vi "2021 Advent puzzle 03b.vi"() -> ()   [LabVIEW 2021]
panel:
  out "x*y":u64
  out "subarray":bool[](array[boolean])
  out "Boolean array 2":bool[][](array[boolean])
  out "number 2":u32
  out "column length 2":i32
  out "Array 2":bool[][](array[boolean])
  out "number":u32
  out "Boolean array":bool[][](array[boolean])
  out "transposed array":bool[][](array[boolean])
  out "Array":bool[][](array[boolean])
  out "Width":i32
  out "column length":i32
  # "11110, 10110, 10111, 10101, 11100, 10000, and 11001."
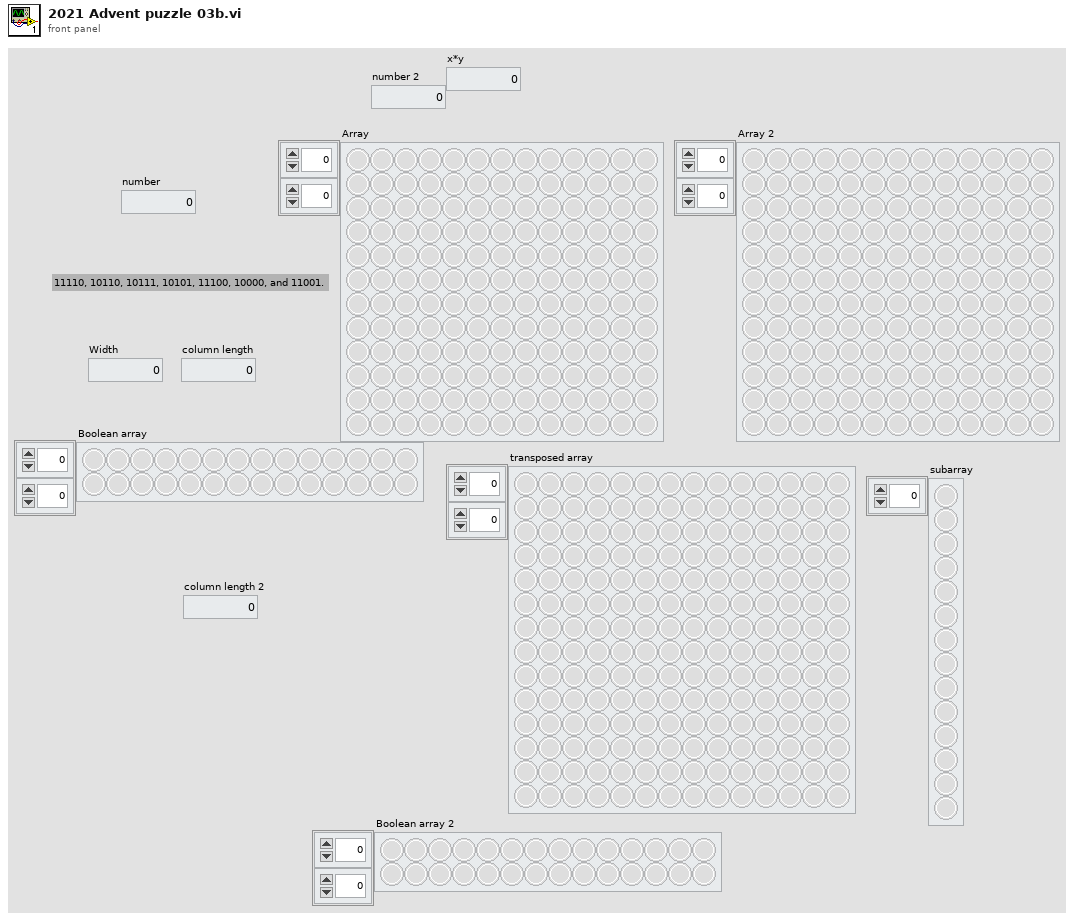
[diagram p1: front panel]
diagram:
  (unwired) "00100\n11110\n10110\n10111\n10101\n01111\n00111\n11100\n10000\n11001\n00010\n01010"
  w6 = "000001100010\n100111011010\n001100011001\n011010001010\n011010101011\n001001110101\n100110001101\n100010010011\n011110000110\n011000110110\n011111111110\n100111110011\n110000100101\n011010011111\n001010011101\n110110001010\n101111110101\n000010101101\n111010111110\n111110001110\n100110111011\n101011010101\n001001000101\n111101000100\n001100000010\n010001100101\n001010011111\n101010010100\n100001110011\n100000111010\n100101010101\n000000101000\n011010100011\n110100111110\n010010011000\n000101000010\n001100011100\n011101000000\n010110111010\n101101100100\n000000010011\n000101001111\n011011100111\n101111100101\n101001101011\n101100010100\n00..."
  # "calc number of 1s per original column\n(number > ((column length div 2 ))generates a true"
  # "determine the number of bits er line"
  n1 = Spreadsheet String To Array(delimiter (Tab)="\n", format string="%b", spreadsheet string=w6, array type (2D Dbl)=i32[] []) -> (array=w14:i32[])
  n2 = Scan From String(format string="%s", input string=w6) -> (output 1=w15:string)  [unwired: 3 in, 3 out]
  n3 = for {
    tunnel: w14 -> [w21] mode=indexing
    tunnel: [w20] -> w11 mode=indexing
    n4 = Number To Boolean Array(number=w21) -> (Boolean array=w20:bool[])
  }
  "transposed array" <- w11
  n5 = String Length(string=w15) -> (length=w7:i32)
  "Width" <- w7
  n6 = Decrement(x=w7) -> (x-1=w8:i32)
  n7 = for {
    N: w7 -> [_]
    shift-right: [w27] -> w13
    shift-left: w11 -> [w28]
    tunnel: w8 -> [w30]
    i -> [w26]
    stop <- w25 stop-if-true
    n8 = Subtract(x=w30, y=w26) -> (x-y=w29:i32)
    n9 = Matrix Size(0:w28) -> (1:w35:i32)  [unwired: 1 out]
    "column length" <- w35
    n10 = Index Array(array=w28, index (col)=w29) -> (element=w31:bool[])  [unwired: 1 in]
    n11 = Boolean To (0,1)(Boolean=w31) -> (0, 1=w32:i16[])
    n12 = Add Array Elements(numeric array=w32) -> (sum=w36:i16)
    n13 = Divide(x=w35, y=2) -> (x/y=w33:dbl)
    n14 = Greater Or Equal?(x=w36, y=w33) -> (x >= y?=w22:bool)
    n15 = for {
      tunnel: w28 -> [w39] mode=indexing
      tunnel: w31 -> [w40] mode=indexing
      tunnel: [w39] -> w27 mode=indexing if=w38
      tunnel: w22 -> [w37]
      n16 = Equal?(x=w40, y=w37) -> (x = y?=w38:bool)
    }
    "Array" <- w27
    n17 = Matrix Size(0:w27) -> (1:w24:i32)  [unwired: 1 out]
    n18 = Equal?(x=w24, y=1) -> (x = y?=w25:bool)
  }
  "Boolean array" <- w13
  n19 = for {
    N: w7 -> [_]
    shift-right: [w46] -> w9
    shift-left: w11 -> [w47]
    tunnel: w8 -> [w49]
    i -> [w45]
    stop <- w44 stop-if-true
    n20 = Subtract(x=w49, y=w45) -> (x-y=w48:i32)
    n21 = Matrix Size(0:w47) -> (1:w54:i32)  [unwired: 1 out]
    "column length 2" <- w54
    n22 = Index Array(array=w47, index (col)=w48) -> (element=w50:bool[])  [unwired: 1 in]
    "subarray" <- w50
    n23 = Boolean To (0,1)(Boolean=w50) -> (0, 1=w51:i16[])
    n24 = Add Array Elements(numeric array=w51) -> (sum=w55:i16)
    n25 = Divide(x=w54, y=2) -> (x/y=w52:dbl)
    n26 = Less?(x=w55, y=w52) -> (x < y?=w41:bool)
    n27 = for {
      tunnel: w47 -> [w58] mode=indexing
      tunnel: w50 -> [w59] mode=indexing
      tunnel: [w58] -> w46 mode=indexing if=w57
      tunnel: w41 -> [w56]
      n28 = Equal?(x=w59, y=w56) -> (x = y?=w57:bool)
    }
    "Array 2" <- w46
    n29 = Matrix Size(0:w46) -> (1:w43:i32)  [unwired: 1 out]
    n30 = Equal?(x=w43, y=1) -> (x = y?=w44:bool)
  }
  "Boolean array 2" <- w9
  n31 = Index Array(array=w9) -> (element=w10:bool[])  [unwired: 2 in]
  n32 = Index Array(array=w13) -> (element=w12:bool[])  [unwired: 2 in]
  n33 = Boolean Array To Number(Boolean array=w10) -> (number=w5:u32)
  "number 2" <- w5
  n34 = Boolean Array To Number(Boolean array=w12) -> (number=w4:u32)
  "number" <- w4
  n35 = To Unsigned Quad Integer(1:w4) -> (0:w2:u64)
  n36 = To Unsigned Quad Integer(1:w5) -> (0:w1:u64)
  n37 = Multiply(x=w2, y=w1) -> (x*y=→"x*y":u64)
